vi "DAQ - WRITE - Double waveform in two channels.vi"(4 "Digital Pause Trigger Pause When":i32(ring)=10192 caption="Pause When" items=["High"=10192, "Low"=10214], 6 "Digital Trigger Source":tag="/Dev1/PFI0" caption="Trigger Source", 7 "Number of Samples":i32=1000, 8 "error in":errorcluster, 9 "data":waveform(dbl)[](array[waveform]), 10 "Sample Rate":dbl=1000.0, 11 "Task/channels in":refnum<k21>) -> (0 "error out":errorcluster, 2 "Actual Sample Rate":dbl=1000.0 format="%0.2f", 3 "task out":refnum<k21>)   [LabVIEW 2017]
uses:
  <vilib>/Utility/error.llb/DialogType.ctl
  <vilib>/DAQmx/write.llb/DAQmx Write (Analog 1D Wfm NChan NSamp).vi
  <vilib>/DAQmx/configure/timing.llb/DAQmx Timing (Sample Clock).vi
  <vilib>/DAQmx/configure/trigger.llb/DAQmx Start Trigger (Digital Edge).vi
  <vilib>/DAQmx/miscellaneous.llb/DAQmx Fill In Error Info.vi
  GLOBAL - FRAME END.vi
  <resource>/objmgr/daqmx.rc
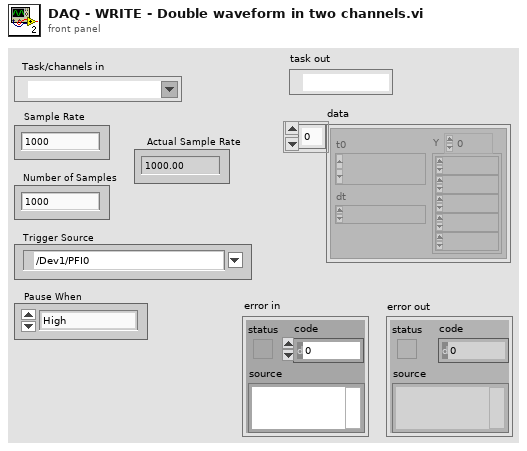
[diagram p1: front panel]
types:
  T1 = typedef "DialogType.ctl" = u16
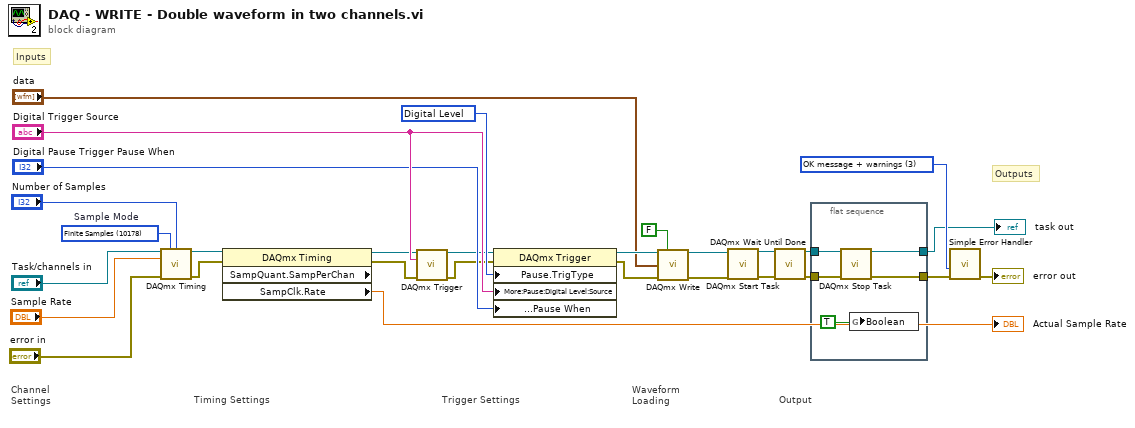
[diagram p0: block diagram]
diagram:
  w14 = 10152 items=["Analog Level"=10101, "Analog Window"=10103, "Digital Level"=10152, "Digital Pattern"=10398, "None"=10230] ("Pause.TrigType")
  w17 = T1 3 items=["no dialog", "OK message", "continue or stop message", "OK message + warnings", "continue/stop + warnings"] ("type of dialog (OK msg:1)")
  w26 = 10178 items=["Finite Samples"=10178, "Continuous Samples"=10123, "Hardware Timed Single Point"=12522]  # Sample Mode
  # "Outputs"
  # "Inputs"
  # "Trigger Settings"
  # "Output"
  # "Waveform \nLoading"
  # "Timing Settings"
  # "Channel \nSettings"
  n1 = call-poly <vilib>:"DAQmx Timing.vi"("task/channels in"="Task/channels in", "sample mode"=w26, "samples per channel"="Number of Samples", "rate"="Sample Rate", "error in"="error in") -> ("task out"=w28:refnum<k21>, "error out"=w27:errorcluster)  [unwired: 9 in]
  n2 = property class="DAQmx Timing" props=["SampQuant.SampPerChan", "SampClk.Rate"](reference=w28, error in=w27) -> (reference out=w15:refnum<k21>, error out=w16:errorcluster, "SampClk.Rate"=→"Actual Sample Rate":dbl)  [unwired: 1 out]
  n3 = call-poly <vilib>:"DAQmx Trigger.vi"("task/channels in"=w15, "source"="Digital Trigger Source", "error in"=w16) -> ("task out"=w12:refnum<k21>, "error out"=w10:errorcluster)  [unwired: 11 in]
  n4 = property class="DAQmx Trigger"(reference=w12, error in=w10, "Pause.TrigType"=w14, "More:Pause:Digital Level:Source"="Digital Trigger Source", "More:Pause:Digital Level:Pause When"="Digital Pause Trigger Pause When") -> (reference out=w11:refnum<k21>, error out=w9:errorcluster)
  n5 = call-poly <vilib>:"DAQmx Write.vi"("task/channels in"=w11, "auto start"=FALSE, "data"="data", "error in"=w9) -> ("task out"=w25:refnum<k21>, "error out"=w24:errorcluster)  [unwired: 9 in, 1 out]
  n6 = call <vilib>:"DAQmx Start Task.vi"("task/channels in"=w25, "error in"=w24) -> ("task out"=w23:refnum<k21>, "error out"=w22:errorcluster)  [unwired: 12 in]
  n7 = call <vilib>:"DAQmx Wait Until Done.vi"("task/channels in"=w23, "error in"=w22) -> ("task out"=w19:refnum<k21>, "error out"=w18:errorcluster)  [unwired: 12 in]
  n8 = flat-sequence {
    tunnel: w19 -> [w34]
    tunnel: w18 -> [w33]
    tunnel: [w32] -> w2
    tunnel: [w31] -> w1
    frame #0 {
      n9 = call <vilib>:"DAQmx Stop Task.vi"("task/channels in"=w34, "error in"=w33) -> ("task out"=w31:refnum<k21>, "error out"=w32:errorcluster)  [unwired: 12 in]
      n10 = global write "GLOBAL - FRAME END.vi" "Boolean"(TRUE) -> ()
    }
  }
  n11 = call <vilib>:"Simple Error Handler.vi"("type of dialog (OK msg:1)"=w17, "error in (no error)"=w2) -> ("error out"=→"error out":errorcluster)  [unwired: 3 in, 4 out]
  "task out" <- w1
